vi "Import Bitmap Demo.vi"() -> ()   [LabVIEW 2013]
doc: "Demonstrate how to use \"Import Bitmap\".\n\n\nGeorge Zou\nhttp://gtoolbox.yeah.net\n\n2002.8."
panel:
  out "new picture":picture
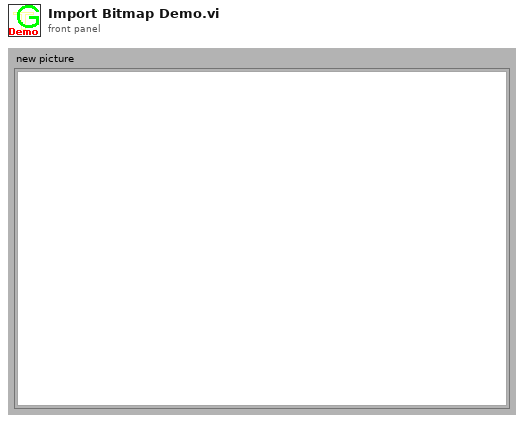
[diagram p1: front panel]
types:
  T1 = cluster{"left":i32, "top":i32, "right":i32, "bottom":i32}
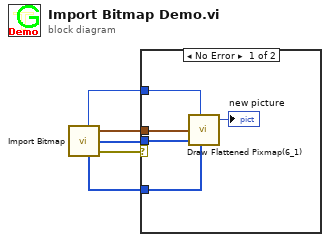
[diagram p0: block diagram]
diagram:
  n1 = call "Import Bitmap.vi"() -> ("color depth"=w5:u8, "rect"=w4:T1, "flattened data"=w3:u8[], "color table"=w2:u32[], "error out"=w1:errorcluster)  [unwired: 5 in]
  n2 = case shown="No Error" w1 {
    tunnel: w5 -> [w10 _]
    tunnel: w4 -> [w9 _]
    tunnel: w3 -> [w8 _]
    tunnel: w2 -> [w7 _]
    frame No Error {
      n3 = call <vilib>:"Draw Flattened Pixmap(6_1).vi"("bit depth(8)"=w10, "rect"=w9, "flattened pixmap data"=w8, "color table"=w7) -> ("new picture"=→"new picture":picture)  [unwired: 5 in]
    }
    frame Error {
    }
  }
